vi "Get Display Text.vi"(8 "error in (no error)":errorcluster, 11 "Element in":refnum<class "Element.lvclass">) -> (0 "error out":errorcluster, 1 "Detail Text":string, 2 "Display Name":string, 3 "Element out":refnum<class "Element.lvclass">)   [LabVIEW 2018, in "VILab.lvlib" / "Element.lvclass"]
uses:
  Element.lvclass
  Element.lvclass/Element.ctl
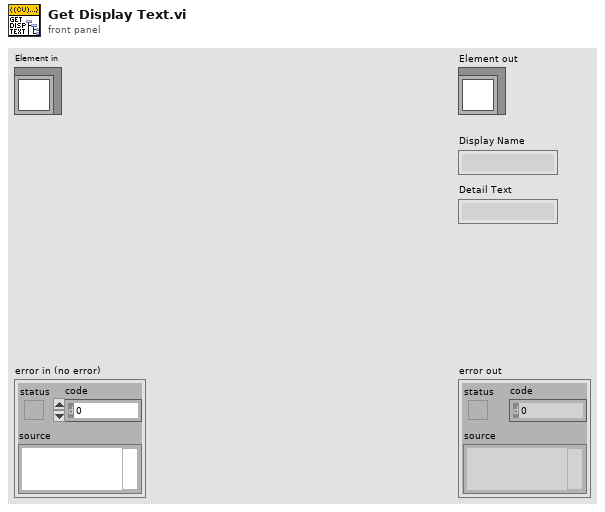
[diagram p1: front panel]
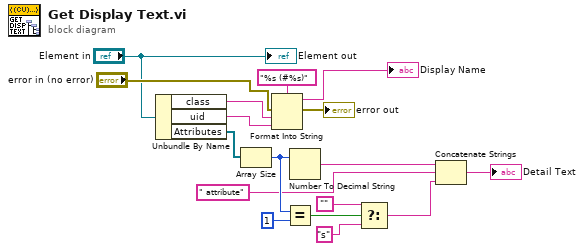
[diagram p0: block diagram]
diagram:
  n1 = Unbundle By Name("Element in") -> ("class"=w16:string, "uid"=w15:string, "Attributes"=w10:refnum<class "Attribute.lvclass">[])
  n2 = Array Size(array=w10) -> (size(s)=w8:i32)
  n3 = Format Into String(format string="%s (#%s)", error in="error in (no error)", w16, w15) -> (resulting string=→"Display Name":string, error out=→"error out":errorcluster)  [unwired: 1 in]
  n4 = Equal?(x=w8, y=1) -> (x = y?=w6:bool)
  n5 = Number To Decimal String(number=w8) -> (decimal integer string=w9:string)  [unwired: 1 in]
  n6 = Select(t="", s=w6, f="s") -> (s? t:f=w2:string)
  n7 = Concatenate Strings(w9, " attribute", w2) -> (→"Detail Text":string)
  "Element out" <- "Element in"
